vi "s4pSave.vi"(8 "error in (no error)":errorcluster caption="错误输入（无错误）", 9 "Channel":string="1", 10 "s4pSavePath":path, 11 "5224A 输入":refnum<class "5224A.lvclass"> caption="DNL_LabVIEW Object in") -> (0 "error out":errorcluster caption="错误输出", 2 "result":bool=TRUE, 3 "5224A 输出":refnum<class "5224A.lvclass"> caption="DNL_LabVIEW Object out")   [LabVIEW 2011, in "5224A.lvclass"]
uses:
  5224A.lvclass
  5224A.lvclass/5224A.ctl
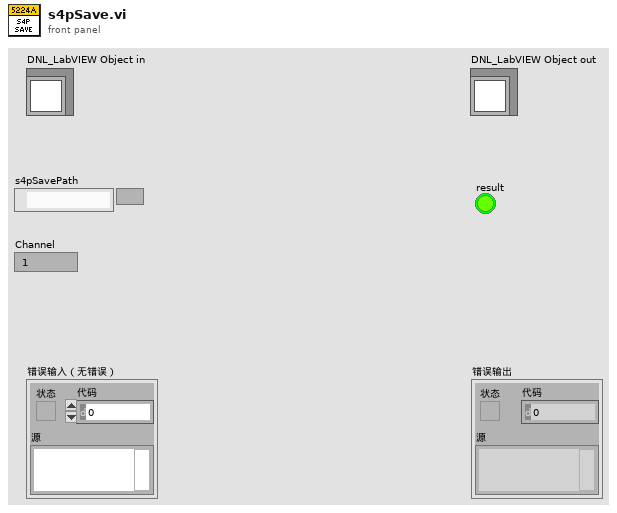
[diagram p1: front panel]
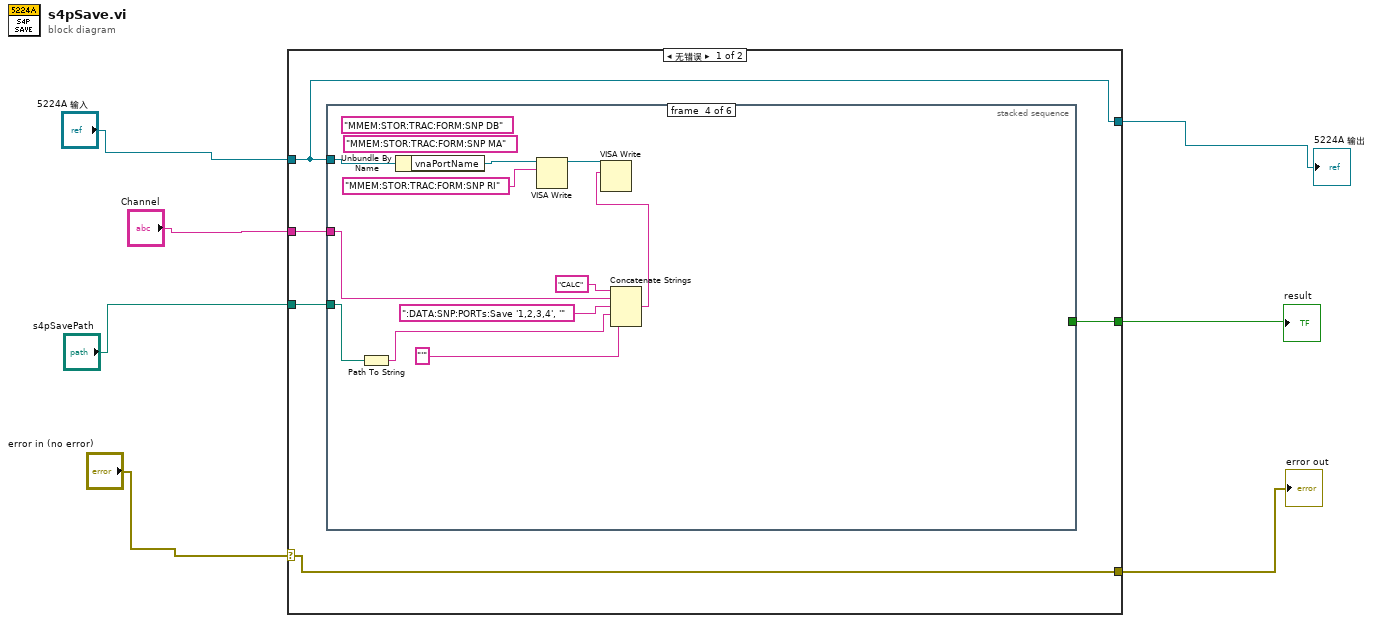
[diagram p0: block diagram]
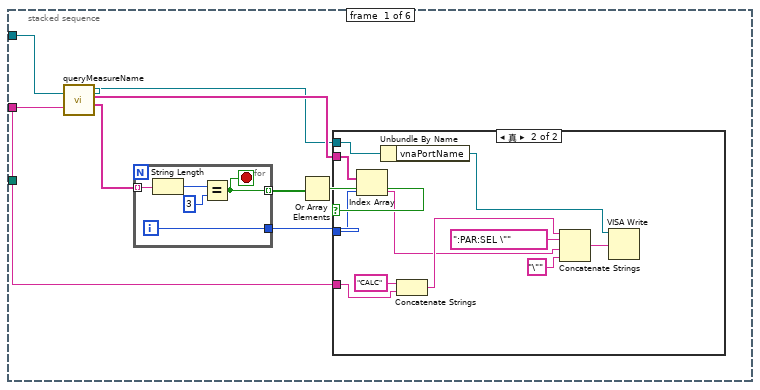
[diagram p2: hidden frame]
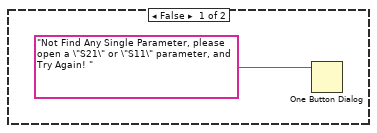
[diagram p3: hidden frame]
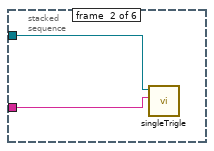
[diagram p4: hidden frame]
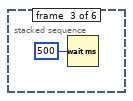
[diagram p5: hidden frame]
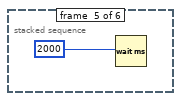
[diagram p6: hidden frame]
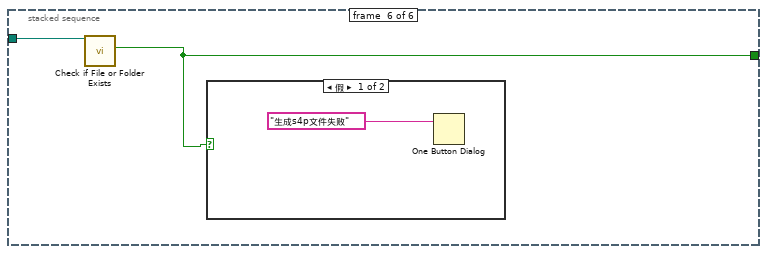
[diagram p7: hidden frame]
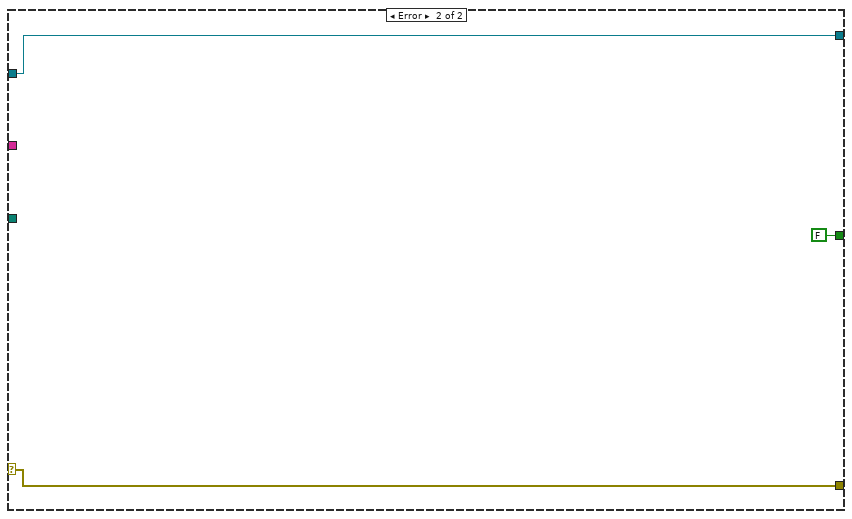
[diagram p9: hidden frame]
diagram:
  n1 = case shown="无错误" "error in (no error)" {
    selector: "error in (no error)" -> [w9 w57]
    tunnel: "5224A 输入" -> [w8 w58]
    tunnel: [w8 w58] -> w6
    tunnel: [w9 w57] -> w1
    tunnel: "Channel" -> [w12 _]
    tunnel: "s4pSavePath" -> [w11 _]
    tunnel: [w10 FALSE ("file or folder exists?")] -> w5
    frame No Error {
      n2 = stacked-sequence {
        tunnel: w8 -> [w20 w39 _ w51 _ _]
        tunnel: w12 -> [w13 w38 _ w43 _ _]
        tunnel: w11 -> [_ _ _ w45 _ w54]
        tunnel: [_ _ _ _ _ w53] -> w10
        frame #0 {
          n3 = call-dynamic "queryMeasureName.vi"("Channel"=w13, "5224A 输入"=w20) -> ("Parameter item"=w18:string[], "Name list"=w16:string[], "5224A 输出"=w14:refnum<class "5224A.lvclass">)  [unwired: 6 in, 1 out]
          n4 = for {
            tunnel: w18 -> [w37] mode=indexing
            tunnel: [w34] -> w19 mode=indexing
            tunnel: [w33] -> w15
            i -> [w33]
            stop <- w34 stop-if-true
            n5 = String Length(string=w37) -> (length=w36:i32)
            n6 = Equal?(x=w36, y=3) -> (x = y?=w34:bool)
          }
          n7 = Or Array Elements(Boolean array=w19) -> (logical OR=w17:bool)
          n8 = case shown="真" w17 {
            tunnel: w16 -> [_ w32]
            tunnel: w15 -> [_ w31]
            tunnel: w14 -> [_ w27]
            tunnel: w13 -> [_ w24]
            frame False {
              n9 = One Button Dialog(message="Not Find Any Single Parameter, please open a \"S21\" or \"S11\" parameter, and Try Again! " ("消息")) -> ()  [unwired: 1 in, 1 out]
            }
            frame True {
              n10 = Index Array(array=w32, index=w31) -> (element=w22:string)
              n11 = Unbundle By Name(w27) -> ("vnaPortName"=w26:refnum<visa-resource-name>)
              n12 = Concatenate Strings("CALC" ("字符串"), w24) -> (w23:string)
              n13 = Concatenate Strings(w23, ":PAR:SEL \"", w22, "\"" ("string")) -> (w28:string)
              n14 = VISA Write(VISA resource name=w26, write buffer=w28) -> ()  [unwired: 1 in, 3 out]
            }
          }
        }
        frame #1 {
          n15 = call-dynamic "singleTrigle.vi"("Channel"=w38, "5224A 输入"=w39) -> ()  [unwired: 8 in, 2 out]
        }
        frame #2 {
          n16 = Wait (ms)(milliseconds to wait=u32 500 ("等待时间（毫秒）")) -> ()  [unwired: 1 out]
        }
        frame #3 {
          (unwired) "MMEM:STOR:TRAC:FORM:SNP DB" ("写入缓冲区")
          (unwired) "MMEM:STOR:TRAC:FORM:SNP MA" ("写入缓冲区")
          n17 = Path To String(path=w45) -> (string=w44:string)
          n18 = Unbundle By Name(w51) -> ("vnaPortName"=w50:refnum<visa-resource-name>)
          n19 = VISA Write(VISA resource name=w50, write buffer="MMEM:STOR:TRAC:FORM:SNP RI" ("写入缓冲区")) -> (VISA resource name out=w48:refnum<visa-resource-name>)  [unwired: 1 in, 2 out]
          n20 = Concatenate Strings("CALC" ("字符串"), w43, ":DATA:SNP:PORTs:Save '1,2,3,4', '" ("写入缓冲区"), w44, "'" ("字符串")) -> (w46:string)
          n21 = VISA Write(VISA resource name=w48, write buffer=w46) -> ()  [unwired: 1 in, 3 out]
        }
        frame #4 {
          n22 = Wait (ms)(milliseconds to wait=u32 2000 ("等待时间（毫秒）")) -> ()  [unwired: 1 out]
        }
        frame #5 {
          n23 = call <vilib>:"Check if File or Folder Exists.vi"("path"=w54) -> ("file or folder exists?"=w53:bool)  [unwired: 8 in, 2 out]
          n24 = case shown="假" w53 {
            frame False {
              n25 = One Button Dialog(message="生成s4p文件失败") -> ()  [unwired: 1 in, 1 out]
            }
            frame True {
            }
          }
        }
      }
    }
    frame Error {
    }
  }
  "error out" <- w1
  "5224A 输出" <- w6
  "result" <- w5
